vi "create dictionary test.vi"() -> ()   [LabVIEW 2013, in "tag bus tests.lvlib"]
uses:
  tag bus tests.lvlib
  dictionary/data dictionary.lvclass
panel:
  out "error out":errorcluster
  in  "count":i32=5000
  out "lookup error":bool
  out "create error":errorcluster
  out "time":dbl
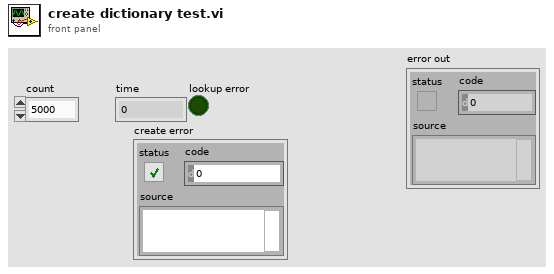
[diagram p1: front panel]
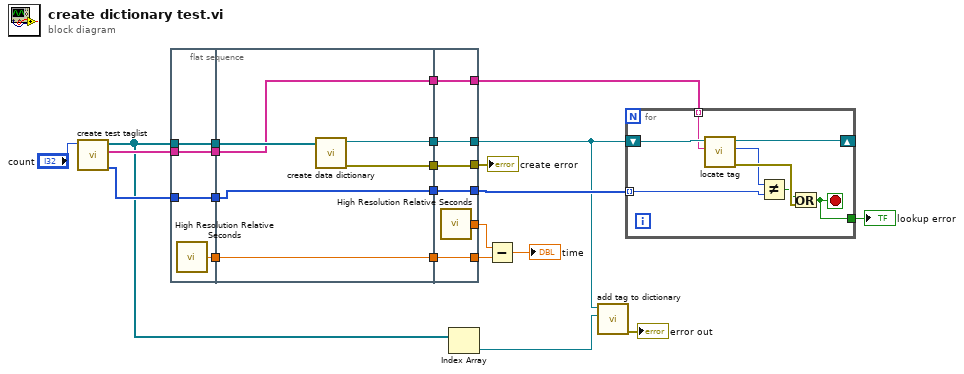
[diagram p0: block diagram]
diagram:
  n1 = call "create test taglist.vi"("count"="count") -> ("indices"=w10:i32[], "names/metadata"=w17:string[], "tags"=w3:refnum<class "tag descriptor.lvclass">[])  [unwired: 7 in, 1 out]
  n2 = flat-sequence {
    tunnel: [w27] -> w22
    tunnel: [w26] -> w18
    tunnel: w3 -> [w26]
    tunnel: w17 -> [w25]
    tunnel: [w25] -> w16
    tunnel: [w24] -> w11
    tunnel: w10 -> [w24]
    tunnel: w22 -> [w33]
    tunnel: [w33] -> w21
    tunnel: w18 -> [w32]
    tunnel: w16 -> [w29]
    tunnel: [w31] -> w15
    tunnel: [w30] -> w14
    tunnel: [w29] -> w13
    tunnel: [w28] -> w12
    tunnel: w11 -> [w28]
    tunnel: [w39] -> w23
    tunnel: w21 -> [w38]
    tunnel: [w38] -> w20
    tunnel: [w37] -> w9
    tunnel: w15 -> [w37]
    tunnel: [w36] -> w4
    tunnel: w14 -> [w36]
    tunnel: [w35] -> w8
    tunnel: w13 -> [w35]
    tunnel: [w34] -> w7
    tunnel: w12 -> [w34]
    frame #0 {
      n3 = call <vilib>:"High Resolution Relative Seconds.vi"() -> ("relative seconds"=w27:dbl)
    }
    frame #1 {
      n4 = call "create data dictionary.vi"("system tags"=w32) -> ("error out"=w31:errorcluster, "data dictionary"=w30:refnum<class "data dictionary.lvclass">)  [unwired: 9 in]
    }
    frame #2 {
      n5 = call <vilib>:"High Resolution Relative Seconds.vi"() -> ("relative seconds"=w39:dbl)
    }
  }
  n6 = Index Array(array=w3) -> (element=w2:refnum<class "tag descriptor.lvclass">)  [unwired: 1 in]
  n7 = Subtract(x=w23, y=w20) -> (x-y=→"time":dbl)
  n8 = call "add tag to dictionary.vi"("system tag"=w2, "data dictionary in"=w4) -> ("error out"=→"error out":errorcluster)  [unwired: 8 in, 1 out]
  n9 = for {
    shift-right: [w41] -> _
    shift-left: w4 -> [w47]
    tunnel: w8 -> [w46] mode=indexing
    tunnel: w7 -> [w42] mode=indexing
    tunnel: [w40] -> w6
    stop <- w40 stop-if-true
    n10 = call "locate tag.vi"("name"=w46, "data dictionary in"=w47) -> ("error out"=w45:errorcluster, "index"=w43:i32, "data dictionary out"=w41:refnum<class "data dictionary.lvclass">)  [unwired: 6 in, 1 out]
    n11 = Not Equal?(x=w43, y=w42) -> (x != y?=w44:bool)
    n12 = Or(x=w44, y=w45) -> (x .or. y?=w40:bool)
  }
  "lookup error" <- w6
  "create error" <- w9
